vi "ShrimpCam_Init.vi"(0 "Camera ID":i32, 1 "Error In":errorcluster) -> (2 "Ref (cam out)":refnum<k24>, 3 "Cam Info":T1={"Bits/Pixel"=8, "Width"=8, "Height Height"=8, "Serial Number "=""}, 4 "Error Out":errorcluster)   [LabVIEW 2018]
uses:
  C:/Users/user/Desktop/Thorcam/uc480DotNet.dll
  Thorcam/uc480DotNet.dll
panel:
  out "Serial Number":string
  out "Height Height":i32=8
  out "Width":i32=8
  out "Bits/Pixel":i32=8
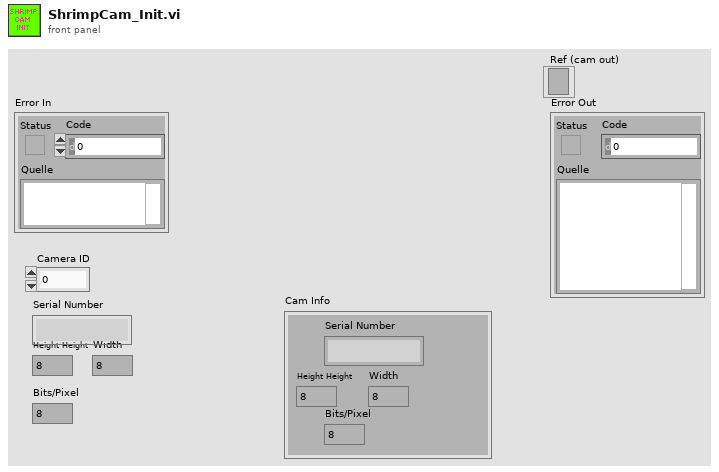
[diagram p1: front panel]
types:
  T1 = cluster{"Bits/Pixel":i32, "Width":i32, "Height Height":i32, "Serial Number ":string}
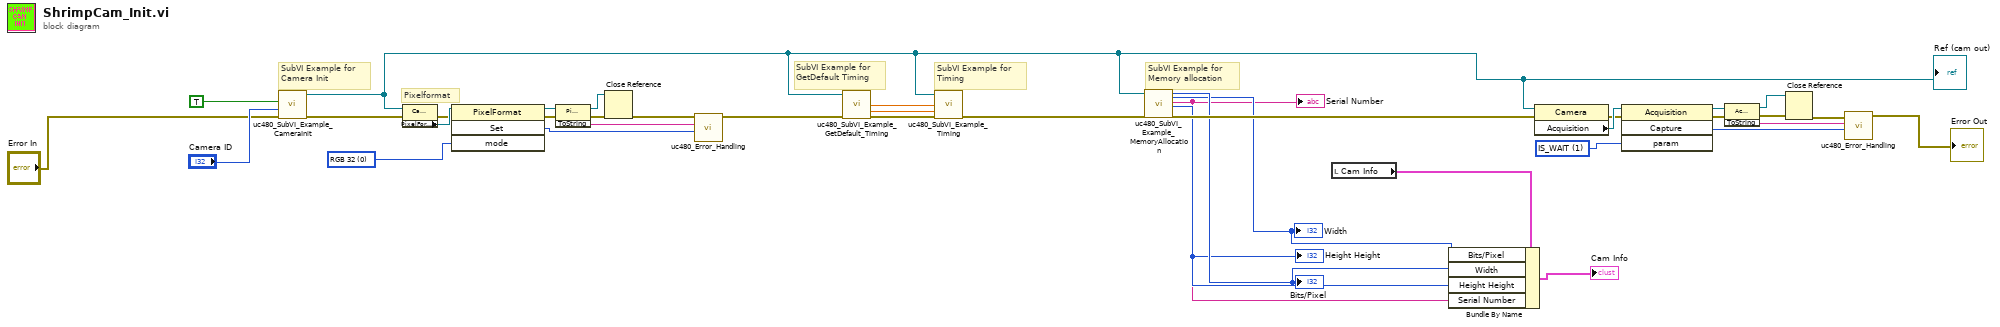
[diagram p0: block diagram]
diagram:
  w18 = 1 items=["IS_DONT_WAIT", "IS_WAIT"] ("Wait")
  w38 = 0 items=["RGB 32"=0, "RGB 24"=1, "Y8 Monochrom"=6] ("Mode")
  # "SubVI Example for \nGetDefault Timing"
  # "SubVI Example for \nMemory allocation"
  # "SubVI Example for \nTiming"
  # "SubVI Example for \nCamera Init"
  # "Pixelformat"
  n1 = call "uc480_SubVI_Example_CameraInit.vi"("Error In"="Error In", "Camera ID"="Camera ID", "Init Camera Flag"=TRUE) -> ("Error Out"=w35:errorcluster, ".NET (Reference)"=w17:refnum<k24>)  [unwired: 7 in]
  "Ref (cam out)" <- w17
  n2 = property class="Camera"(reference=w17, error in=w35) -> (error out=w36:errorcluster, "PixelFormat"=w37:refnum<k24>)  [unwired: 1 out]
  n3 = invoke class="PixelFormat" method="Set"(reference=w37, error in=w36, "mode"=w38) -> (reference out=w33:refnum<k24>, error out=w29:errorcluster, "Set"=w32:i32)  [unwired: 1 in, 1 out]
  n4 = invoke class="PixelFormat" method="ToString"(reference=w33, error in=w29) -> (reference out=w13:refnum<k24>, error out=w14:errorcluster, "ToString"=w34:string)  [unwired: 1 in]
  n5 = Close Reference(reference=w13, error in (no error)=w14) -> (error out=w12:errorcluster)
  n6 = call "uc480_Error_Handling.vi"("Error Code"=w32, "Error String"=w34, "Error In"=w12) -> ("Error Out"=w27:errorcluster)  [unwired: 8 in]
  n7 = call "uc480_SubVI_Example_GetDefault_Timing.vi"(".NET (Reference)"=w17, "Error In"=w27) -> ("Exposure time"=w25:dbl, "Framerate"=w26:dbl, "Error Out"=w15:errorcluster)  [unwired: 10 in, 1 out]
  n8 = call "uc480_SubVI_Example_Timing.vi"(".NET (Reference)"=w17, "Exposure time"=w25, "Framerate"=w26, "Error In"=w15) -> ("Error Out"=w28:errorcluster)  [unwired: 8 in, 3 out]
  n9 = call "uc480_SubVI_Example_MemoryAllocation.vi"(".NET (Reference)"=w17, "Error In"=w28) -> ("Bits/Pixel 2"=w5:i32, "Width"=w4:i32, "Serial Number"=w2:string, "Height"=w3:i32, "Error Out"=w16:errorcluster)  [unwired: 13 in]
  "Bits/Pixel" <- w5
  "Width" <- w4
  "Height Height" <- w3
  "Serial Number" <- w2
  n10 = local read "Cam Info"() -> (w6:T1)
  n11 = Bundle By Name(cluster=w6, "Bits/Pixel"=w5, "Width"=w4, "Height Height"=w3, "Serial Number"=w2) -> (→"Cam Info":T1)
  n12 = property class="Camera"(reference=w17, error in=w16) -> (error out=w23:errorcluster, "Acquisition"=w24:refnum<k24>)  [unwired: 1 out]
  n13 = invoke class="Acquisition" method="Capture"(reference=w24, error in=w23, "param"=w18) -> (reference out=w20:refnum<k24>, error out=w21:errorcluster, "Capture"=w19:i32)  [unwired: 1 in, 1 out]
  n14 = invoke class="Acquisition" method="ToString"(reference=w20, error in=w21) -> (reference out=w9:refnum<k24>, error out=w11:errorcluster, "ToString"=w22:string)  [unwired: 1 in]
  n15 = Close Reference(reference=w9, error in (no error)=w11) -> (error out=w10:errorcluster)
  n16 = call "uc480_Error_Handling.vi"("Error Code"=w19, "Error String"=w22, "Error In"=w10) -> ("Error Out"=→"Error Out":errorcluster)  [unwired: 8 in]
